vi "Main.vi"() -> ()   [LabVIEW 2015]
doc: "This template is for the Queued Message Handler design pattern.\n\nThe Event Handling Loop generates messages based on user interface actions.\n\nThe Message Handling Loop processes messages generated by the Event Handling Loop, or by other messages. The messages are string values, so new messages can be added easily to the Message Cases case structure in the Message Handling Loop. Each message cluster can also provide an optional value for Message Data, which is a variant that can be converted to whatever message-specific data is required."
uses:
  controls/UI Data.ctl
  support/Boiler System Globals.vi
  support/Message Queue/Message Queue.lvlib
  support/User Event - Stop/User Event - Stop.lvlib
panel:
  out "Display <Replace Me>":string
  in  "Do Something Else <Replace Me>":bool
  in  "Do Something <Replace Me>":bool
  in  "Stop Button":bool
  # "These controls have associated \"Value Changed\" events configured in the Event Structure on the diagram.\n\nReplace them (and reconfigure the Event Structure) with the controls you need for your application."
  # "This template is for the Queued Message Handler design pattern.\n\nSee the block diagram for more information on how to use this template."
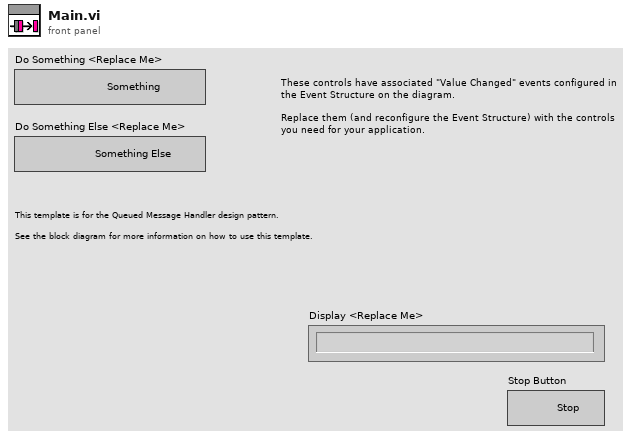
[diagram p1: front panel]
types:
  T1 = typedef "UI Data.ctl" = cluster{"Boolean <Replace Me>":bool, "String <Replace Me>":string, "Numeric <Replace Me>":dbl, "Do Something Ref":refnum<vi>, "Do Something Else Ref":refnum<vi>, "Data Display Ref":refnum<vi>, "Stop Button Ref":refnum<vi>}
  T2 = typedef "Message Queue.lvlib/All Message Queues.ctl" = cluster{"MHL":refnum<queue>, "Boiler Controler":refnum<queue>}
  T3 = enum32{"invalid app kind", "Development System", "Run Time System", "Student Edition", "Embedded LabVIEW", "Evaluation", "Custom"}
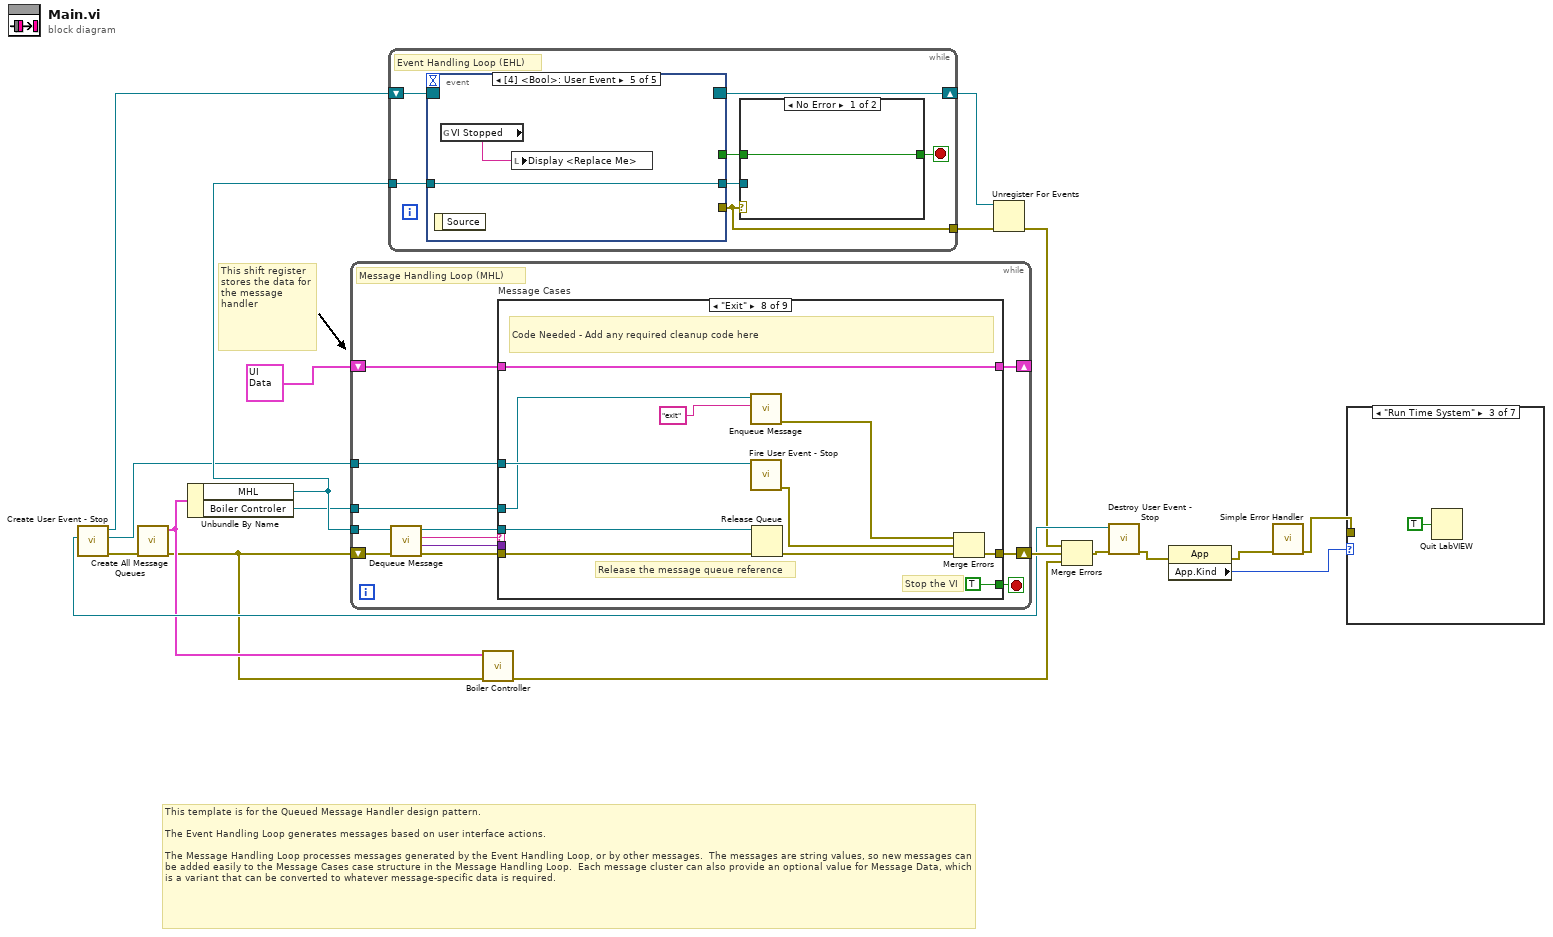
[diagram p0: block diagram]
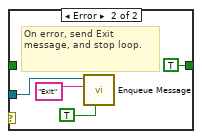
[diagram p8: hidden frame]
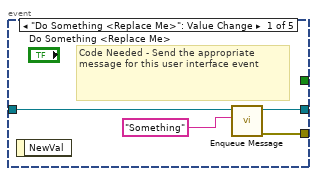
[diagram p9: hidden frame]
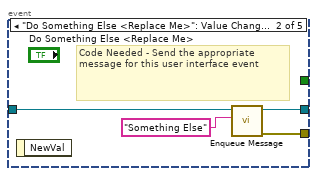
[diagram p10: hidden frame]
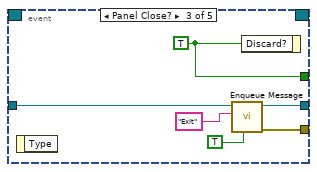
[diagram p11: hidden frame]
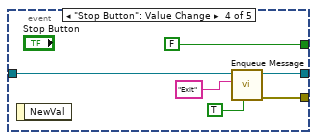
[diagram p12: hidden frame]
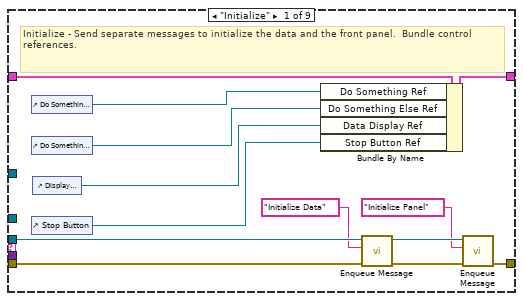
[diagram p13: hidden frame]
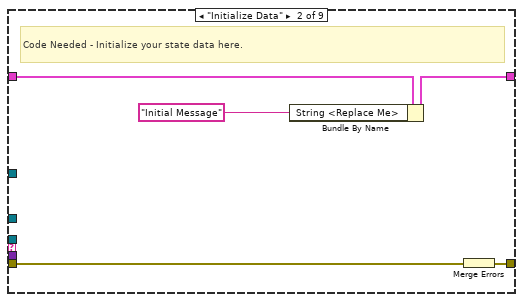
[diagram p14: hidden frame]
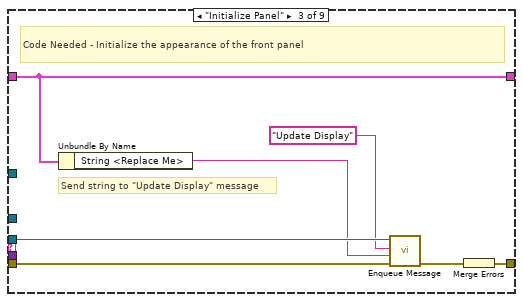
[diagram p15: hidden frame]
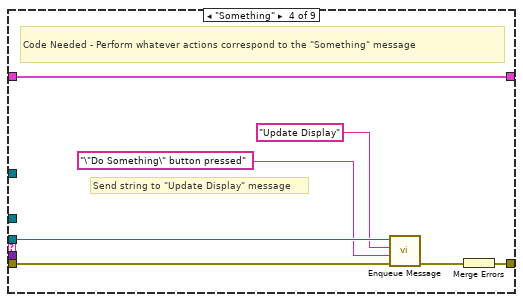
[diagram p16: hidden frame]
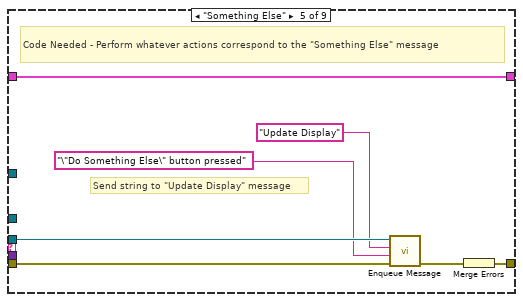
[diagram p17: hidden frame]
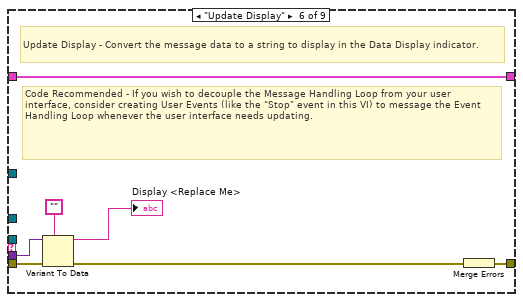
[diagram p18: hidden frame]
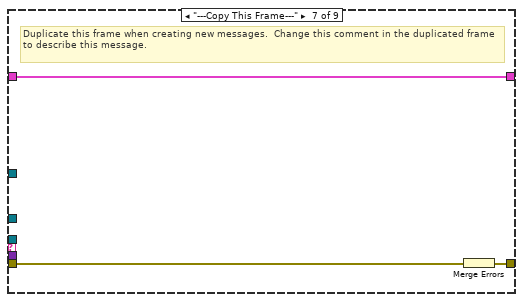
[diagram p19: hidden frame]
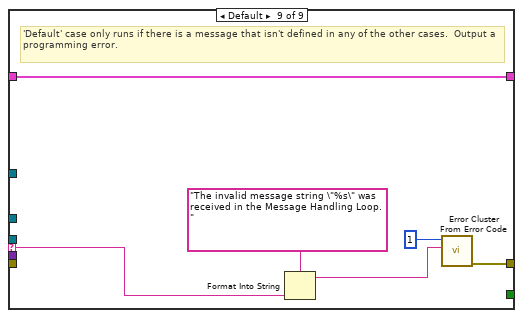
[diagram p20: hidden frame]
diagram:
  # "This template is for the Queued Message Handler design pattern.\n\nThe Event Handling Loop generates messages based on user interface actions.\n\nThe Message Handling Loop processes messages generated by the Event Handling Loop, or by other messages.  The messages are string values, so new messages can be added easily to the Message Cases case structure in the Message Handling Loop.  Each message cluster can also provide an optional value for Message Data, which is a variant that can be converted to whatever message-specific data is required."
  # "This shift register\nstores the data for the message handler"
  n1 = call "Create User Event - Stop.vi"() -> ("error out"=w16:errorcluster, "User bool - Stop"=w14:refnum<user-event>, "Event Registration Refnum"=w9:refnum<event-registration>)  [unwired: 9 in]
  n2 = call "Create All Message Queues.vi"("error in (no error)"=w16) -> ("error out"=w7:errorcluster, "Message Queues out"=w8:T2)  [unwired: 9 in]
  n3 = Unbundle By Name(w8) -> ("MHL"=w17:refnum<queue>, "Boiler Controler"=w5:refnum<queue>)
  n4 = while {
    tunnel: w17 -> [w20]
    shift-right: [w29] -> _
    shift-left: T1 {"Boolean <Replace Me>"=TRUE, "String <Replace Me>"="", "Numeric <Replace Me>"=0.0, "Do Something Ref"=refnum, "Do Something Else Ref"=refnum, "Data Display Ref"=refnum, "Stop Button Ref"=refnum} ("Data Cluster") -> [w30]
    tunnel: w14 -> [w26]
    shift-right: [w27] -> w18
    shift-left: w7 -> [w25]
    tunnel: w5 -> [w19]
    stop <- w28 stop-if-true
    # "Message Handling Loop (MHL)"
    n5 = call "Dequeue Message.vi"("error in (no error)"=w25, "Message Queue"=w20) -> ("error out"=w24:errorcluster, "Message Data"=w22:variant, "Message"=w23:string, "dup Message Queue"=w21:refnum<queue>)  [unwired: 6 in]
    n6 = case "Message Cases" shown="\"Exit\"" w23 {
      selector: w23 -> [_ _ _ _ _ _ _ _ w94]
      tunnel: w21 -> [w39 _ w52 w58 w65 _ _ w90 _]
      tunnel: w24 -> [w42 w48 w53 w60 w67 w74 w79 w85 _]
      tunnel: [w43 w44 w54 w61 w68 w75 w77 w86 w92] -> w27
      tunnel: w30 -> [w36 w47 w55 w62 w69 w76 w78 w89 w96]
      tunnel: [w35 w46 w55 w62 w69 w76 w78 w89 w96] -> w29
      tunnel: [_ _ _ _ _ _ _ TRUE _] -> w28
      tunnel: w22 -> [_ _ _ _ _ w73 _ _ _]
      tunnel: w26 -> [_ _ _ _ _ _ _ w84 _]
      tunnel: w19 -> [_ _ _ _ _ _ _ w82 _]
      frame "Initialize" {
        # "Initialize - Send separate messages to initialize the data and the front panel.  Bundle control references."
        n7 = control-ref of="Do Something <Replace Me>"() -> (w34:refnum<vi>)
        n8 = control-ref of="Do Something Else <Replace Me>"() -> (w33:refnum<vi>)
        n9 = control-ref of="Stop Button"() -> (w31:refnum<vi>)
        n10 = control-ref of="Display <Replace Me>"() -> (w32:refnum<vi>)
        n11 = Bundle By Name(cluster=w36, "Do Something Ref"=w34, "Do Something Else Ref"=w33, "Data Display Ref"=w32, "Stop Button Ref"=w31) -> (w35:T1)
        n12 = call "Enqueue Message.vi"("error in (no error)"=w42, "Message"="Initialize Data", "Message Queue"=w39) -> ("error out"=w41:errorcluster, "dup Message Queue"=w40:refnum<queue>)  [unwired: 7 in]
        n13 = call "Enqueue Message.vi"("error in (no error)"=w41, "Message"="Initialize Panel", "Message Queue"=w40) -> ("error out"=w43:errorcluster)  [unwired: 7 in, 1 out]
      }
      frame "Initialize Data" {
        # "Code Needed - Initialize your state data here."
        n14 = Bundle By Name(cluster=w47, "String <Replace Me>"="Initial Message" ("Initial Message")) -> (w46:T1)
        n15 = Merge Errors(w48) -> (w44:errorcluster)
      }
      frame "Initialize Panel" {
        # "Send string to \"Update Display\" message"
        # "Code Needed - Initialize the appearance of the front panel"
        n16 = Unbundle By Name(w55) -> ("String <Replace Me>"=w49:string)
        n17 = call "Enqueue Message.vi"("error in (no error)"=w53, "Message Data"=w49, "Message"="Update Display", "Message Queue"=w52) -> ("error out"=w51:errorcluster)  [unwired: 6 in, 1 out]
        n18 = Merge Errors(w51) -> (w54:errorcluster)
      }
      frame "Something" {
        # "Send string to \"Update Display\" message"
        # "Code Needed - Perform whatever actions correspond to the \"Something\" message"
        n19 = call "Enqueue Message.vi"("error in (no error)"=w60, "Message Data"="\"Do Something\" button pressed" ("\"Do Something\" button pressed"), "Message"="Update Display", "Message Queue"=w58) -> ("error out"=w59:errorcluster)  [unwired: 6 in, 1 out]
        n20 = Merge Errors(w59) -> (w61:errorcluster)
      }
      frame "Something Else" {
        # "Send string to \"Update Display\" message"
        # "Code Needed - Perform whatever actions correspond to the \"Something Else\" message"
        n21 = call "Enqueue Message.vi"("error in (no error)"=w67, "Message Data"="\"Do Something Else\" button pressed" ("\"Do Something Else\" button pressed"), "Message"="Update Display", "Message Queue"=w65) -> ("error out"=w66:errorcluster)  [unwired: 6 in, 1 out]
        n22 = Merge Errors(w66) -> (w68:errorcluster)
      }
      frame "Update Display" {
        # "Code Recommended - If you wish to decouple the Message Handling Loop from your user interface, consider creating User Events (like the \"Stop\" event in this VI) to message the Event Handling Loop whenever the user interface needs updating."
        # "Update Display - Convert the message data to a string to display in the Data Display indicator."
        n23 = Variant To Data(error in=w74, type="", Variant=w73) -> (data=→"Display <Replace Me>":string, error out=w71:errorcluster)
        n24 = Merge Errors(w71) -> (w75:errorcluster)
      }
      frame "---Copy This Frame---" {
        # "Duplicate this frame when creating new messages.  Change this comment in the duplicated frame to describe this message."
        n25 = Merge Errors(w79) -> (w77:errorcluster)
      }
      frame "Exit" {
        # "Stop the VI"
        # "Release the message queue reference"
        # "Code Needed - Add any required cleanup code here"
        n26 = call "Enqueue Message.vi"("Message"="exit", "Message Queue"=w82) -> ("error out"=w80:errorcluster)  [unwired: 8 in, 1 out]
        n27 = call "Fire User Event - Stop.vi"("User Event - Stop"=w84) -> ("error out"=w83:errorcluster)  [unwired: 10 in]
        n28 = Release Queue(queue=w90, error in (no error)=w85) -> (error out=w87:errorcluster)  [unwired: 1 in, 2 out]
        n29 = Merge Errors(w80, w83, w87) -> (w86:errorcluster)
      }
      frame Default {
        # "'Default' case only runs if there is a message that isn't defined in any of the other cases.  Output a programming error."
        n30 = Format Into String(format string="The invalid message string \"%s\" was received in the Message Handling Loop." ("Unknown Message Error Text"), w94) -> (resulting string=w91:string)  [unwired: 2 in, 1 out]
        n31 = call <vilib>:"Error Cluster From Error Code.vi"("error message (\"\")"=w91, "error code (0)"=1) -> ("error out"=w92:errorcluster)  [unwired: 7 in]
      }
    }
  }
  n32 = while {
    tunnel: w17 -> [w103]
    tunnel: [w99] -> w12
    shift-right: [w98] -> w11
    shift-left: w9 -> [w97]
    stop <- w101 stop-if-true
    # "Event Handling Loop (EHL)"
    n33 = event shown="[4] <Bool>: User Event" {
      selector: w97 -> [_ _ _ _ _]
      dyn-events: [_ _ _ _ _] -> w98
      timeout: _ -> [_ _ _ _ _]
      tunnel: [_ _ w122 FALSE ("Discard?") _] -> w102
      tunnel: w103 -> [w112 w116 w121 w128 w130]
      tunnel: [w111 w114 w120 w127 _] -> w99
      tunnel: [w110 w115 w119 w125 w130] -> w100
      event "Do Something <Replace Me>": Value Change {
        # "Code Needed - Send the appropriate message for this user interface event"
        n34 = event-data() -> ()  [unwired: 1 in, 1 out]
        n35 = call "Enqueue Message.vi"("Message"="Something", "Message Queue"=w112) -> ("error out"=w111:errorcluster, "dup Message Queue"=w110:refnum<queue>)  [unwired: 8 in]
      }
      event "Do Something Else <Replace Me>": Value Change {
        # "Code Needed - Send the appropriate message for this user interface event"
        n36 = event-data() -> ()  [unwired: 1 in, 1 out]
        n37 = call "Enqueue Message.vi"("Message"="Something Else", "Message Queue"=w116) -> ("error out"=w114:errorcluster, "dup Message Queue"=w115:refnum<queue>)  [unwired: 8 in]
      }
      event Panel Close? {
        w122 = TRUE ("Discard?")
        n38 = event-data() -> ()  [unwired: 1 in, 1 out]
        n39 = call "Enqueue Message.vi"("Priority Message? (F)"=TRUE, "Message"="Exit", "Message Queue"=w121) -> ("error out"=w120:errorcluster, "dup Message Queue"=w119:refnum<queue>)  [unwired: 7 in]
        n40 = event-data("Discard?"=w122) -> ()  [unwired: 1 in, 1 out]
      }
      event "Stop Button": Value Change {
        n41 = event-data() -> ()  [unwired: 1 in, 1 out]
        n42 = call "Enqueue Message.vi"("Priority Message? (F)"=TRUE, "Message"="Exit", "Message Queue"=w128) -> ("error out"=w127:errorcluster, "dup Message Queue"=w125:refnum<queue>)  [unwired: 7 in]
      }
      event User Event {
        n43 = event-data() -> ()  [unwired: 1 in, 1 out]
        n44 = global read "Boiler System Globals.vi" "VI Stopped"() -> (w129:string)
        n45 = local write "Display <Replace Me>"(w129) -> ()
      }
    }
    n46 = case shown="No Error" w99 {
      tunnel: [w104 TRUE ("Discard?")] -> w101
      tunnel: w102 -> [w104 _]
      tunnel: w100 -> [_ w107]
      frame No Error {
      }
      frame Error {
        # "On error, send Exit message, and stop loop."
        n47 = call "Enqueue Message.vi"("Priority Message? (F)"=TRUE, "Message"="Exit", "Message Queue"=w107) -> ()  [unwired: 7 in, 2 out]
      }
    }
  }
  n48 = call "Boiler Controller.vi"("Error In"=w7, "Message Queues"=w8) -> ("Error Out"=w6:errorcluster)  [unwired: 9 in]
  n49 = Unregister For Events(event registration refnum=w11, error in=w12) -> (error out=w13:errorcluster)
  n50 = Merge Errors(w13, w18, w6) -> (w15:errorcluster)
  n51 = call "Destroy User Event - Stop.vi"("error in (no error)"=w15, "User Event - Stop"=w14) -> ("error out"=w4:errorcluster)  [unwired: 9 in]
  n52 = property class="App"(error in=w4) -> (error out=w3:errorcluster, "App.Kind"=w1:T3)  [unwired: 1 in, 1 out]
  n53 = call <vilib>:"Simple Error Handler.vi"("error in (no error)"=w3) -> ("error out"=w2:errorcluster)  [unwired: 4 in, 4 out]
  n54 = case shown="\"Run Time System\"" w1 {
    tunnel: w2 -> [_ _ _ _ _ _ _]
    frame "invalid app kind", Default {
    }
    frame "Development System" {
    }
    frame "Run Time System" {
      n55 = Quit LabVIEW(quit? (T)=TRUE) -> ()
    }
    frame "Student Edition" {
    }
    frame "Embedded LabVIEW" {
    }
    frame "Evaluation" {
    }
    frame "Custom" {
    }
  }
